vi "Clone Template Main.vi"() -> ()   [LabVIEW 2020, in "Template Tool.lvlib"]
uses:
  Template Tool.lvlib
  Queue Cluster.ctl
  Consumer State.ctl
  Consumer Data.ctl
  3a5bffab-33ac-43cc-aa37-910ccd41f3ad.vi
panel:
  in  "cancelling":string="\nCANCELLING\n\nThis may take a moment."
  out "Build Time (m:ss)":string
  in  "stop":bool
  out "message":string
  out "Progress":u8(slide) scale=0.0..100.0
  in  "start":bool
  in  "cancel":bool
  in  "Enter Destination Directory":path
  in  "Enter Custom Device Name":string="My New Comms"
  # "Instructions:\n1. Run this VI.\n2. Enter a Custom Device Name and Destination Directory.\n3. Press Start."
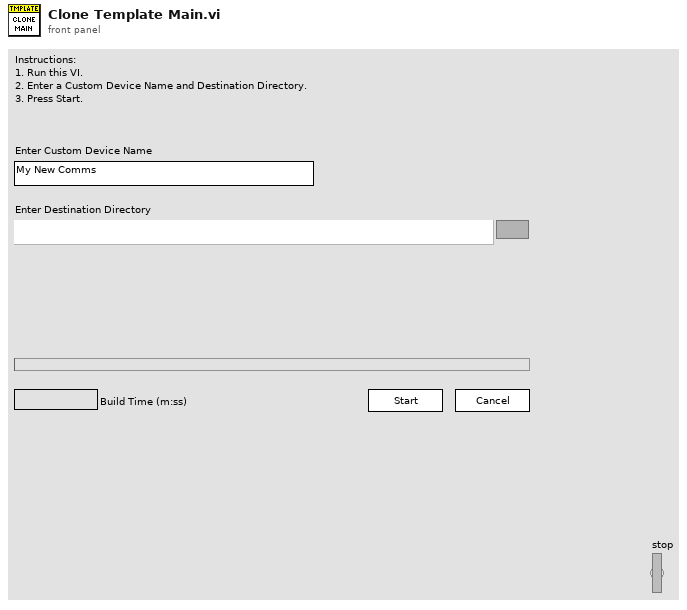
[diagram p1: front panel]
types:
  T1 = typedef "Template Tool.lvlib/Consumer Data.ctl" = cluster{"xml name":string, "CD name":string, "CD lvproj name":string, "CD support lvproj name":string, "custom device path":path, "progress":u8, "relative LVLIB folders":path[], "Public Docs CD path":path, "custom device lvproj path":path}
  T2 = typedef "Template Tool.lvlib/Queue Cluster.ctl" = cluster{"state":T3, "data":variant}
  T3 = typedef "Template Tool.lvlib/Consumer State.ctl" = enum16{"Init", "Cancel", "Copy Source", "Build Original Support PPLs", "Update Help Files", "Edit Page VIs Help CHM Constant", "Includes Folder AutoPopulate Off", "Replace VI & XML GUIDs", "Edit Paths in XML", "Edit CD Name in XML", "Edit VI Constants", "Edit Build Spec Destinations", "Delete Test Folders", "Create & Replace Support LVLIB Copies to Temp", "Create & Replace Support LVLIB Copies to Original", "Rename LVLIBS in Support LVPROJ File", "Update Support Build Specs and Build", "Replace Project PPLs", "Includes Folder AutoPopulate On", "Create & Replace LVLIB Copies to Temp", "Create & Replace LVLIB Copies to Original", "Rename LVLIBS in LVPROJ File", "Rename LLBs", "Update Build Specs and Build", "Finish"}
  T4 = cluster{"Enter Custom Device Name":string, "Enter Destination Directory":path}
  T5 = enum16{"Rename Original to Temp", "Rename Temp to Original"}
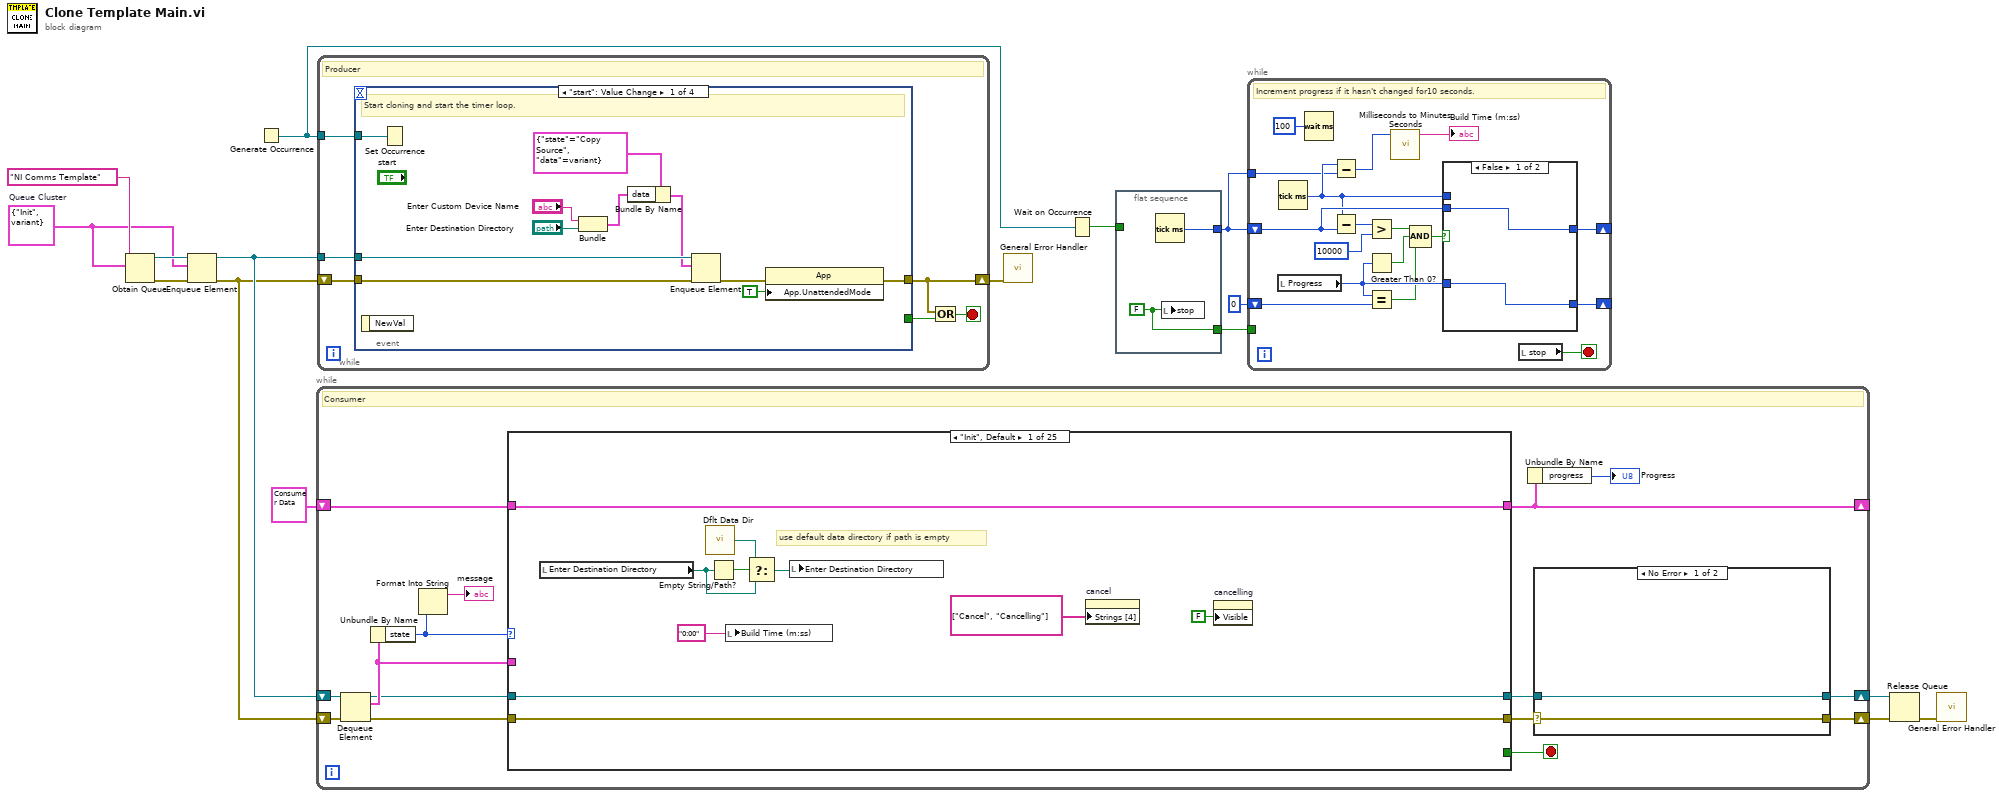
[diagram p0: block diagram]
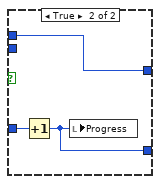
[diagram p2: hidden frame]
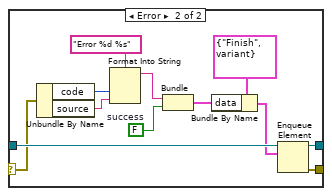
[diagram p3: hidden frame]
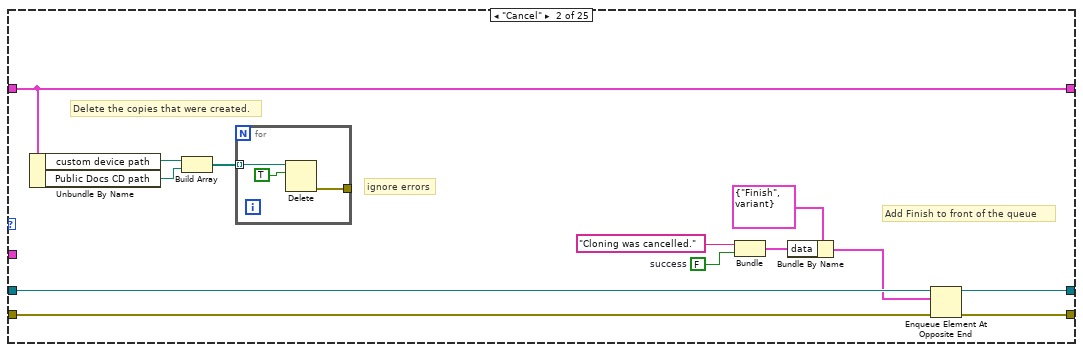
[diagram p4: hidden frame]
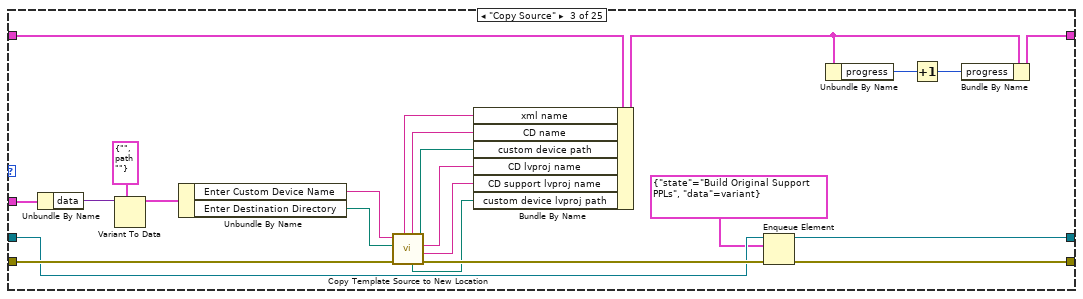
[diagram p5: hidden frame]
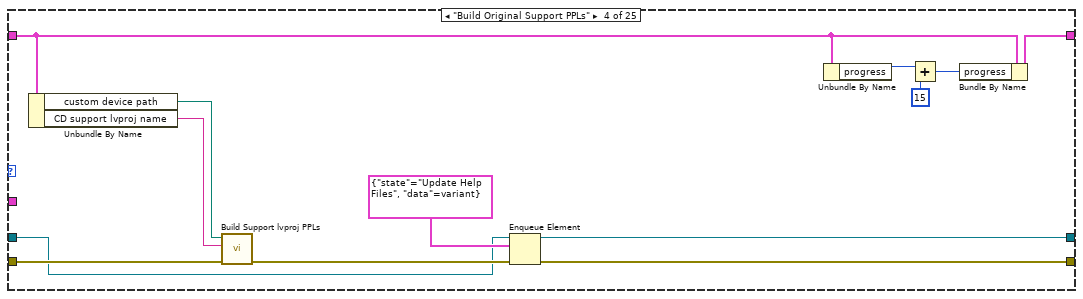
[diagram p6: hidden frame]
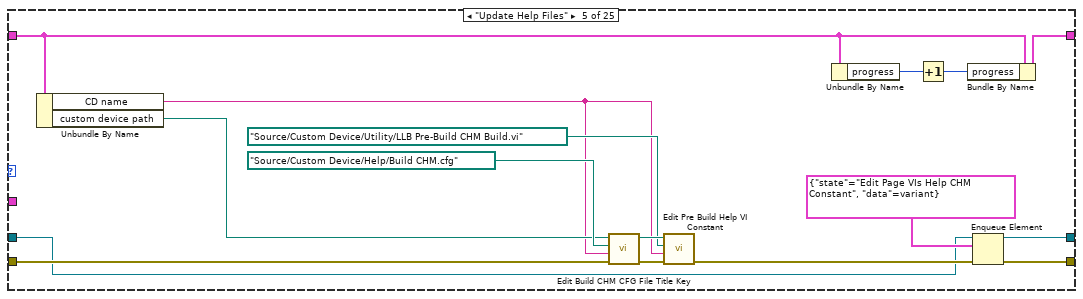
[diagram p7: hidden frame]
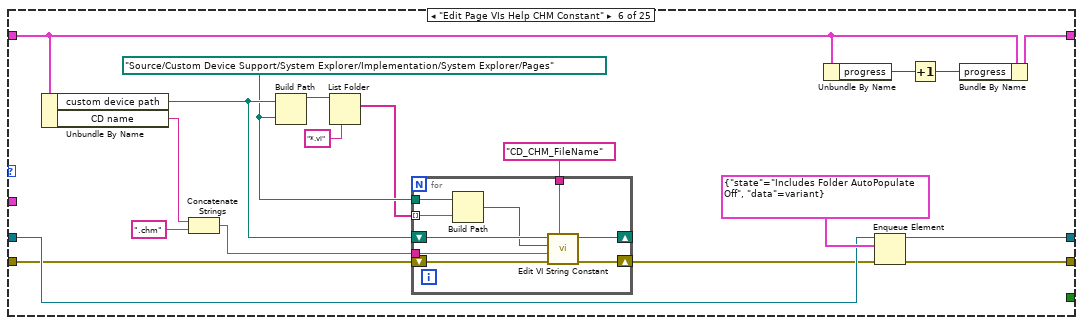
[diagram p8: hidden frame]
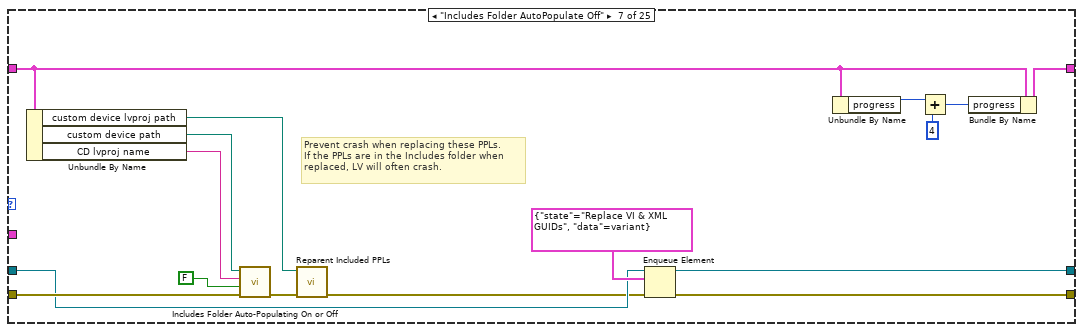
[diagram p9: hidden frame]
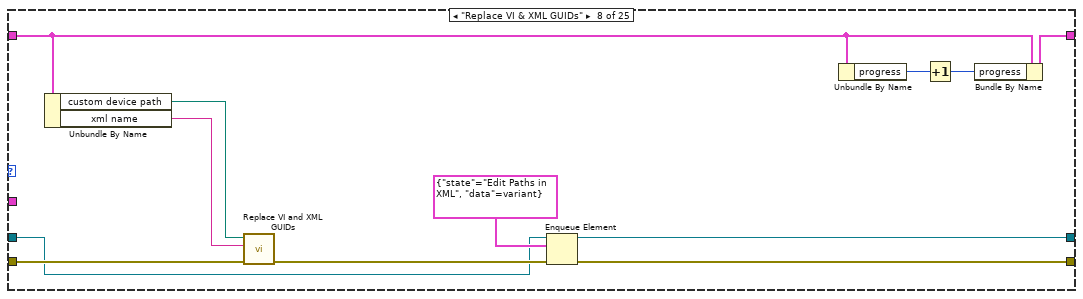
[diagram p10: hidden frame]
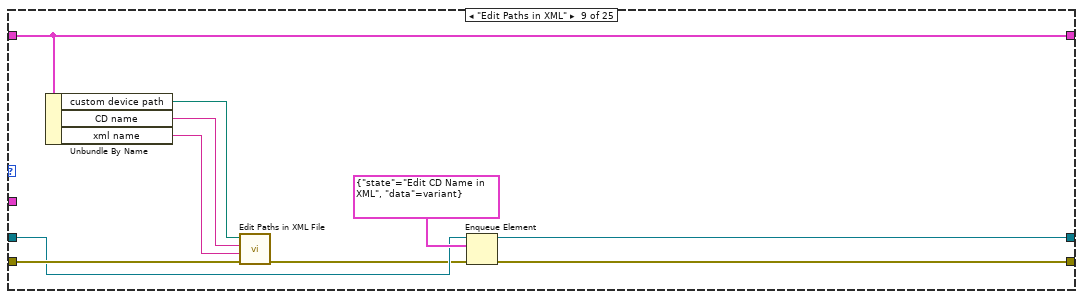
[diagram p11: hidden frame]
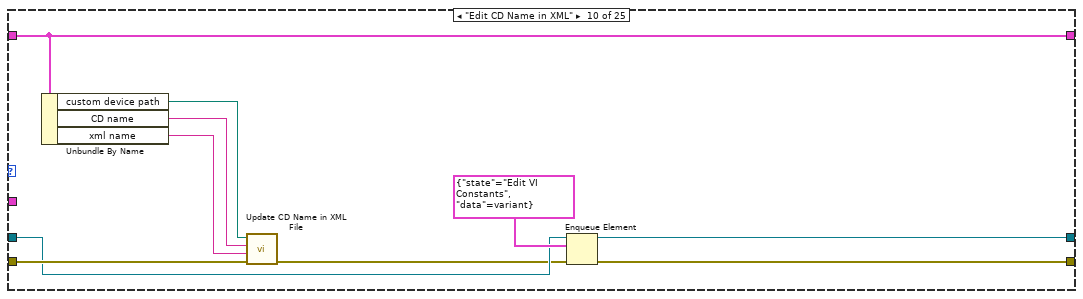
[diagram p12: hidden frame]
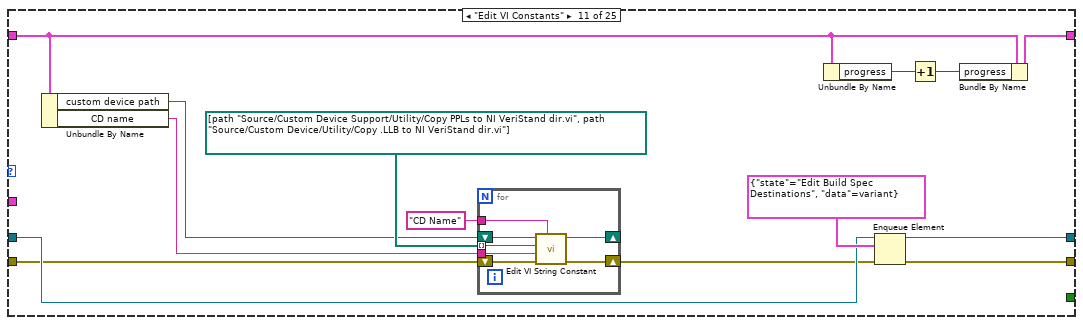
[diagram p13: hidden frame]
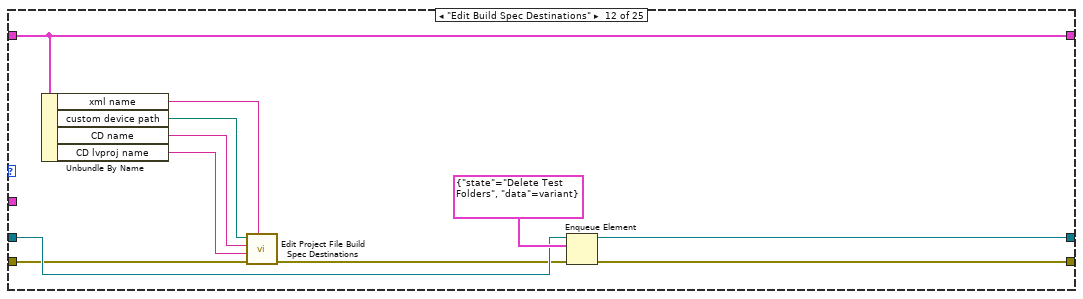
[diagram p14: hidden frame]
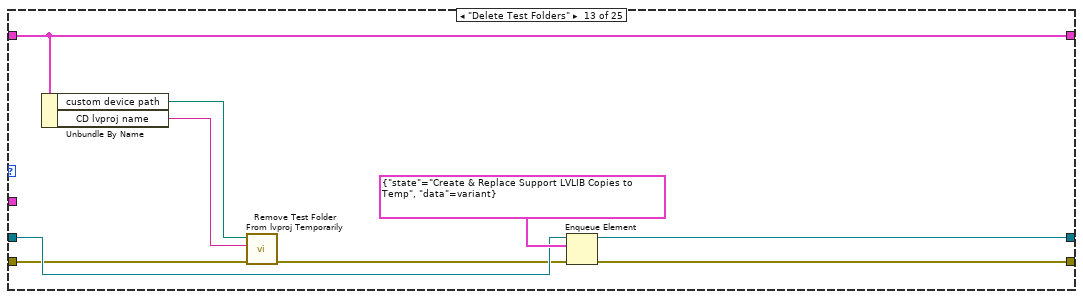
[diagram p15: hidden frame]
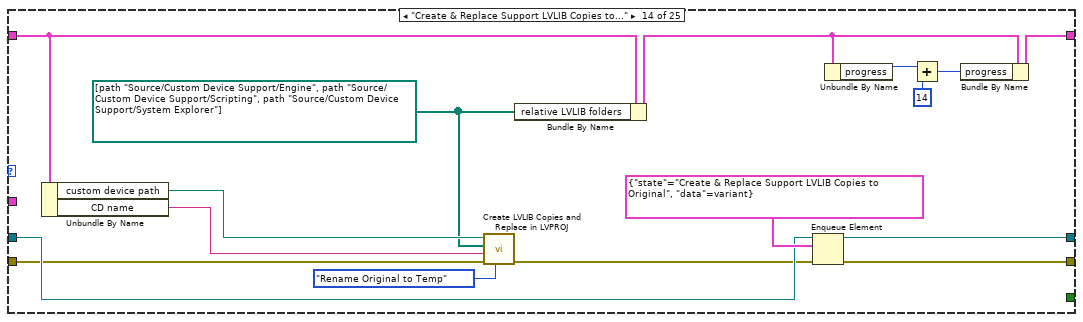
[diagram p16: hidden frame]
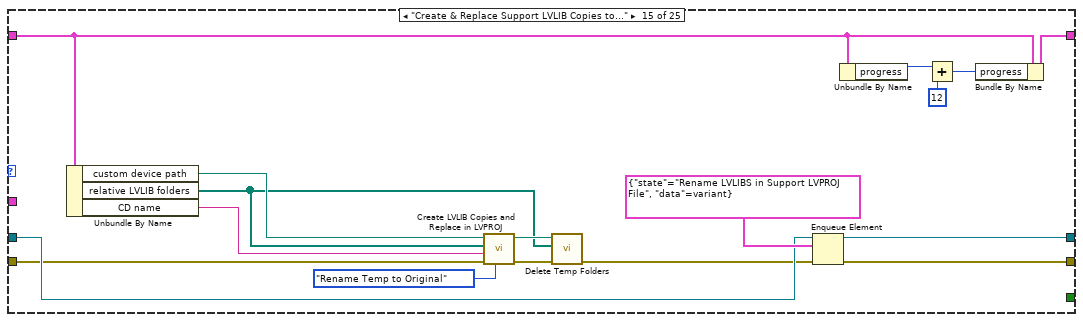
[diagram p17: hidden frame]
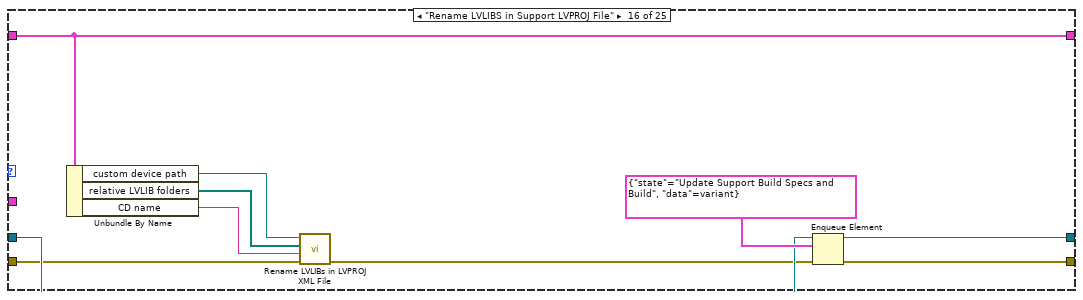
[diagram p18: hidden frame]
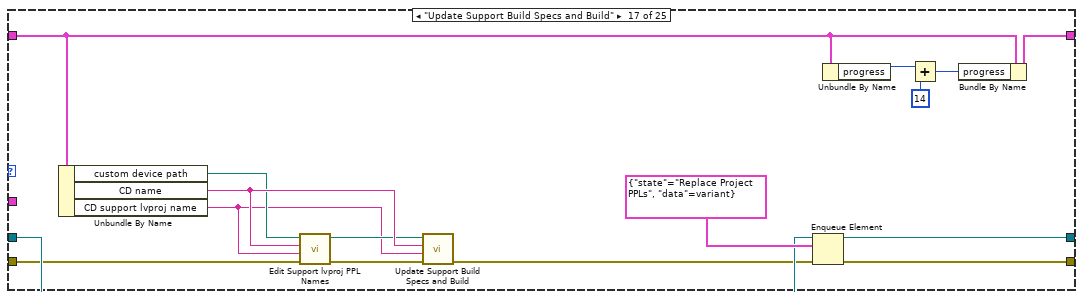
[diagram p19: hidden frame]
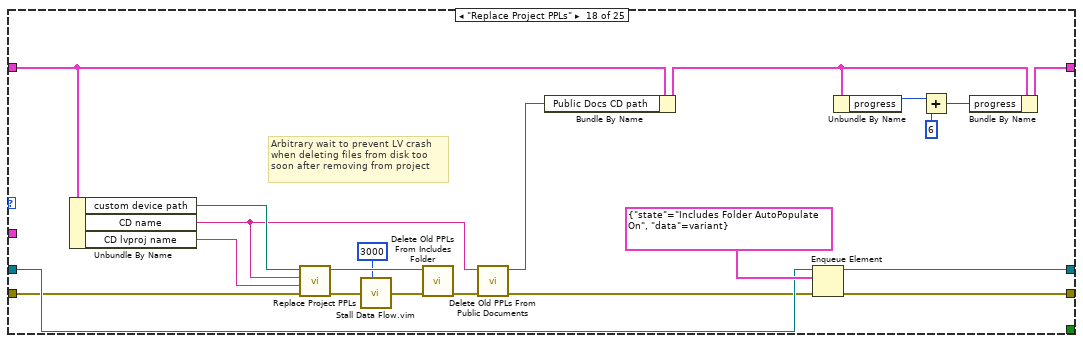
[diagram p20: hidden frame]
diagram:
  w12 = T2 {"state"=enum."Init", "data"=variant}  # Queue Cluster
  n1 = Obtain Queue(name (unnamed)="NI Comms Template", element data type=w12) -> (queue out=w15:refnum<queue>, error out=w14:errorcluster)  [unwired: 3 in, 1 out]
  n2 = Enqueue Element(queue=w15, element=w12, error in (no error)=w14) -> (queue out=w13:refnum<queue>, error out=w11:errorcluster)  [unwired: 1 in, 1 out]
  n3 = Generate Occurrence() -> (w2:refnum<k4>)
  n4 = while {
    shift-right: [w20] -> w9
    shift-left: w11 -> [w28]
    shift-right: [w23] -> _
    shift-left: T1 {"xml name"="", "CD name"="", "CD lvproj name"="", "CD support lvproj name"="", "custom device path"=path "", "progress"=0, "relative LVLIB folders"=[], "Public Docs CD path"=path "", "custom device lvproj path"=path ""} ("Consumer Data") -> [w29]
    shift-right: [w18] -> w8
    shift-left: w13 -> [w31]
    stop <- w17 stop-if-true
    # "Consumer"
    n5 = Dequeue Element(queue=w31, error in (no error)=w28) -> (queue out=w26:refnum<queue>, element=w30:T2, error out=w27:errorcluster)  [unwired: 1 in, 1 out]
    n6 = Unbundle By Name(w30) -> ("state"=w25:T3)
    n7 = Format Into String(w25) -> (resulting string=→"message":string)  [unwired: 3 in, 1 out]
    n8 = case shown="\"Init\", Default" w25 {
      tunnel: w30 -> [_ _ w94 _ _ _ _ _ _ _ _ _ _ _ _ _ _ _ _ _ _ _ _ _ w429]
      tunnel: [_ _ _ _ _ _ _ _ _ _ _ _ _ _ _ _ _ _ _ _ _ _ _ _ w420] -> w17
      tunnel: w27 -> [w50 w68 w93 w106 w119 w139 w167 w179 w188 w199 w209 w227 w236 w252 w270 w277 w295 w314 w334 w342 w368 w379 w389 w414 w418]
      tunnel: [w50 w67 w80 w103 w114 w137 w162 w174 w180 w190 w206 w221 w232 w246 w262 w279 w296 w317 w328 w348 w360 w381 w393 w415 w419] -> w21
      tunnel: w29 -> [w54 w58 w87 w98 w109 w134 w156 w169 w189 w198 w203 w231 w240 w256 w258 w280 w285 w308 w322 w354 w356 w373 w394 w410 w422]
      tunnel: [w54 w58 w73 w97 w108 w133 w155 w168 w189 w198 w202 w231 w240 w241 w257 w280 w284 w307 w321 w343 w355 w372 w394 w409 w422] -> w23
      tunnel: w26 -> [w55 w66 w79 w102 w112 w141 w161 w173 w183 w193 w212 w229 w238 w254 w272 w282 w298 w319 w327 w352 w370 w383 w396 w417 w427]
      tunnel: [w55 w65 w77 w101 w113 w140 w160 w172 w182 w192 w211 w228 w237 w253 w271 w281 w297 w318 w326 w351 w369 w382 w395 w416 w427] -> w19
      frame "Init", Default {
        # "use default data directory if path is empty"
        n9 = local read "Enter Destination Directory"() -> (w46:path)
        n10 = call <vilib>:"Dflt Data Dir.vi"() -> ("App:Default Data Directory"=w48:path)
        n11 = Empty String/Path?(string/path=w46) -> (empty?=w49:bool)
        n12 = local write "Build Time (m:ss)"("0:00" ("Build Time (m:s)")) -> ()
        n13 = Select(t=w48, s=w49, f=w46) -> (s? t:f=w47:path)
        n14 = local write "Enter Destination Directory"(w47) -> ()
        n15 = property on="cancel" class="Bool"("Strings [4]"=string[] ["Cancel", "Cancelling"]) -> ()  [unwired: 2 in, 2 out]
        n16 = property on="cancelling" class="Str"("Visible"=FALSE) -> ()  [unwired: 2 in, 2 out]
      }
      frame "Cancel" {
        w59 = FALSE  # success
        # "ignore errors"
        # "Add Finish to front of the queue"
        # "Delete the copies that were created."
        n17 = Unbundle By Name(w58) -> ("custom device path"=w64:path, "Public Docs CD path"=w56:path)
        n18 = Build Array(w64, w56) -> (w57:path[])
        n19 = for {
          tunnel: w57 -> [w71] mode=indexing
          tunnel: [w69] -> _
          n20 = Delete(path (use dialog)=w71, entire hierarchy (F)=TRUE) -> (error out=w69:errorcluster)  [unwired: 3 in, 2 out]
        }
        n21 = Bundle("dialog message"="Cloning was cancelled.", "success"=w59) -> (w60:cluster{"dialog message":string, "success":bool})  [unwired: 1 in]
        n22 = Bundle By Name(cluster=T2 {"state"=enum."Finish", "data"=variant} ("Queue Cluster"), "data"=w60) -> (w62:T2)
        n23 = Enqueue Element At Opposite End(queue=w66, element=w62, error in (no error)=w68) -> (queue out=w65:refnum<queue>, error out=w67:errorcluster)  [unwired: 1 in, 1 out]
      }
      frame "Copy Source" {
        n24 = Unbundle By Name(w94) -> ("data"=w92:variant)
        n25 = Variant To Data(type=T4 {"Enter Custom Device Name"="", "Enter Destination Directory"=path ""} ("output cluster"), Variant=w92) -> (data=w90:T4)  [unwired: 1 in, 1 out]
        n26 = Unbundle By Name(w90) -> ("Enter Custom Device Name"=w89:string, "Enter Destination Directory"=w88:path)
        n27 = call "Copy Template Source to New Location.vi"("error in"=w93, "destination directory (default data directory if empty)"=w88, "custom device name"=w89) -> ("error out"=w81:errorcluster, "CD support lvproj name"=w82:string, "CD lvproj name"=w83:string, "custom device path out"=w84:path, "custom device lvproj path"=w72:path, "CD name"=w85:string, "xml name"=w86:string)  [unwired: 2 in]
        n28 = Bundle By Name(cluster=w87, "xml name"=w86, "CD name"=w85, "custom device path"=w84, "CD lvproj name"=w83, "CD support lvproj name"=w82, "custom device lvproj path"=w72) -> (w74:T1)
        n29 = Enqueue Element(queue=w79, element=T2 {"state"=enum."Build Original Support PPLs", "data"=variant} ("Queue Cluster"), error in (no error)=w81) -> (queue out=w77:refnum<queue>, error out=w80:errorcluster)  [unwired: 1 in, 1 out]
        n30 = Unbundle By Name(w74) -> ("progress"=w76:u8)
        n31 = Increment(x=w76) -> (x+1=w75:u8)
        n32 = Bundle By Name(cluster=w74, "progress"=w75) -> (w73:T1)
      }
      frame "Build Original Support PPLs" {
        n33 = Unbundle By Name(w98) -> ("custom device path"=w107:path, "CD support lvproj name"=w100:string)
        n34 = call "Build Support lvproj PPLs.vi"("error in"=w106, "CD support lvproj name"=w100, "custom device path"=w107) -> ("error out"=w104:errorcluster)  [unwired: 7 in, 1 out]
        n35 = Enqueue Element(queue=w102, element=T2 {"state"=enum."Update Help Files", "data"=variant} ("Queue Cluster"), error in (no error)=w104) -> (queue out=w101:refnum<queue>, error out=w103:errorcluster)  [unwired: 1 in, 1 out]
        n36 = Unbundle By Name(w98) -> ("progress"=w96:u8)
        n37 = Add(x=w96, y=u8 15) -> (x+y=w99:u8)
        n38 = Bundle By Name(cluster=w98, "progress"=w99) -> (w97:T1)
      }
      frame "Update Help Files" {
        n39 = Unbundle By Name(w109) -> ("CD name"=w117:string, "custom device path"=w118:path)
        n40 = call "Edit Build CHM CFG File Title Key.vi"("error in"=w119, "CD name"=w117, "relative path of CFG file to edit"=path "Source/Custom Device/Help/Build CHM.cfg" ("relative path of VI to edit"), "custom device path"=w118) -> ("error out"=w121:errorcluster, "custom device path out"=w122:path)  [unwired: 6 in]
        n41 = call "Edit Pre Build Help VI Constant.vi"("error in"=w121, "CD name"=w117, "relative path of VI to edit"=path "Source/Custom Device/Utility/LLB Pre-Build CHM Build.vi", "custom device path"=w122) -> ("error out"=w115:errorcluster)  [unwired: 6 in, 1 out]
        n42 = Unbundle By Name(w109) -> ("progress"=w111:u8)
        n43 = Increment(x=w111) -> (x+1=w110:u8)
        n44 = Bundle By Name(cluster=w109, "progress"=w110) -> (w108:T1)
        n45 = Enqueue Element(queue=w112, element=T2 {"state"=enum."Edit Page VIs Help CHM Constant", "data"=variant} ("Queue Cluster"), error in (no error)=w115) -> (queue out=w113:refnum<queue>, error out=w114:errorcluster)  [unwired: 1 in, 1 out]
      }
      frame "Edit Page VIs Help CHM Constant" {
        w128 = path "Source/Custom Device Support/System Explorer/Implementation/System Explorer/Pages" ("name or relative path")
        n46 = Unbundle By Name(w134) -> ("custom device path"=w131:path, "CD name"=w124:string)
        n47 = Concatenate Strings(w124, ".chm" ("string")) -> (w125:string)
        n48 = Build Path(base path=w131, name or relative path=w128) -> (appended path=w130:path)
        n49 = List Folder(path=w130, pattern="*.vi") -> (filenames=w127:string[])  [unwired: 2 in, 3 out]
        n50 = for {
          shift-right: [w149] -> w138
          shift-left: w139 -> [w150]
          shift-right: [w148] -> _
          shift-left: w131 -> [w151]
          tunnel: w125 -> [w147]
          tunnel: "CD_CHM_FileName" ("CD name") -> [w146]
          tunnel: w128 -> [w145]
          tunnel: w127 -> [w144] mode=indexing
          n51 = Build Path(base path=w145, name or relative path=w144) -> (appended path=w143:path)
          n52 = call "Edit VI String Constant.vi"("string label"=w146, "error in"=w150, "new value"=w147, "relative path of VI to edit"=w143, "custom device path"=w151) -> ("error out"=w149:errorcluster, "custom device path out"=w148:path)  [unwired: 5 in]
        }
        n53 = Unbundle By Name(w134) -> ("progress"=w136:u8)
        n54 = Enqueue Element(queue=w141, element=T2 {"state"=enum."Includes Folder AutoPopulate Off", "data"=variant} ("Queue Cluster"), error in (no error)=w138) -> (queue out=w140:refnum<queue>, error out=w137:errorcluster)  [unwired: 1 in, 1 out]
        n55 = Increment(x=w136) -> (x+1=w135:u8)
        n56 = Bundle By Name(cluster=w134, "progress"=w135) -> (w133:T1)
      }
      frame "Includes Folder AutoPopulate Off" {
        # "Prevent crash when replacing these PPLs.\nIf the PPLs are in the Includes folder when\nreplaced, LV will often crash."
        n57 = Unbundle By Name(w156) -> ("custom device lvproj path"=w152:path, "custom device path"=w166:path, "CD lvproj name"=w165:string)
        n58 = call "Includes Folder Auto-Populating On or Off.vi"("error in"=w167, "auto-populate (ON)"=FALSE, "CD lvproj name"=w165, "custom device path"=w166) -> ("error out"=w154:errorcluster)  [unwired: 6 in, 1 out]
        n59 = call "Reparent Included PPLs.vi"("error in"=w154, "custom device project"=w152) -> ("error out"=w153:errorcluster)  [unwired: 9 in]
        n60 = Enqueue Element(queue=w161, element=T2 {"state"=enum."Replace VI & XML GUIDs", "data"=variant} ("Queue Cluster"), error in (no error)=w153) -> (queue out=w160:refnum<queue>, error out=w162:errorcluster)  [unwired: 1 in, 1 out]
        n61 = Unbundle By Name(w156) -> ("progress"=w158:u8)
        n62 = Add(x=w158, y=u8 4) -> (x+y=w159:u8)
        n63 = Bundle By Name(cluster=w156, "progress"=w159) -> (w155:T1)
      }
      frame "Replace VI & XML GUIDs" {
        n64 = Unbundle By Name(w169) -> ("custom device path"=w178:path, "xml name"=w177:string)
        n65 = call "Replace VI and XML GUIDs.vi"("error in"=w179, "xml name"=w177, "custom device path"=w178) -> ("error out"=w175:errorcluster)  [unwired: 7 in, 1 out]
        n66 = Enqueue Element(queue=w173, element=T2 {"state"=enum."Edit Paths in XML", "data"=variant} ("Queue Cluster"), error in (no error)=w175) -> (queue out=w172:refnum<queue>, error out=w174:errorcluster)  [unwired: 1 in, 1 out]
        n67 = Unbundle By Name(w169) -> ("progress"=w171:u8)
        n68 = Increment(x=w171) -> (x+1=w170:u8)
        n69 = Bundle By Name(cluster=w169, "progress"=w170) -> (w168:T1)
      }
      frame "Edit Paths in XML" {
        n70 = Unbundle By Name(w189) -> ("custom device path"=w187:path, "CD name"=w186:string, "xml name"=w185:string)
        n71 = call "Edit Paths in XML File.vi"("error in"=w188, "xml name"=w185, "CD name"=w186, "custom device path"=w187) -> ("error out"=w181:errorcluster)  [unwired: 5 in, 2 out]
        n72 = Enqueue Element(queue=w183, element=T2 {"state"=enum."Edit CD Name in XML", "data"=variant} ("Queue Cluster"), error in (no error)=w181) -> (queue out=w182:refnum<queue>, error out=w180:errorcluster)  [unwired: 1 in, 1 out]
      }
      frame "Edit CD Name in XML" {
        n73 = Unbundle By Name(w198) -> ("custom device path"=w197:path, "CD name"=w196:string, "xml name"=w195:string)
        n74 = call "Update CD Name in XML File.vi"("error in"=w199, "xml name"=w195, "CD name"=w196, "custom device path"=w197) -> ("error out"=w191:errorcluster)  [unwired: 6 in, 1 out]
        n75 = Enqueue Element(queue=w193, element=T2 {"state"=enum."Edit VI Constants", "data"=variant} ("Queue Cluster"), error in (no error)=w191) -> (queue out=w192:refnum<queue>, error out=w190:errorcluster)  [unwired: 1 in, 1 out]
      }
      frame "Edit VI Constants" {
        n76 = Unbundle By Name(w203) -> ("custom device path"=w208:path, "CD name"=w201:string)
        n77 = for {
          shift-right: [w218] -> w207
          shift-left: w209 -> [w219]
          tunnel: path[] [path "Source/Custom Device Support/Utility/Copy PPLs to NI VeriStand dir.vi", path "Source/Custom Device/Utility/Copy .LLB to NI VeriStand dir.vi"] -> [w217] mode=indexing
          shift-right: [w216] -> _
          shift-left: w208 -> [w220]
          tunnel: w201 -> [w215]
          tunnel: "CD Name" ("CD name") -> [w214]
          n78 = call "Edit VI String Constant.vi"("string label"=w214, "error in"=w219, "new value"=w215, "relative path of VI to edit"=w217, "custom device path"=w220) -> ("error out"=w218:errorcluster, "custom device path out"=w216:path)  [unwired: 5 in]
        }
        n79 = Unbundle By Name(w203) -> ("progress"=w205:u8)
        n80 = Enqueue Element(queue=w212, element=T2 {"state"=enum."Edit Build Spec Destinations", "data"=variant} ("Queue Cluster"), error in (no error)=w207) -> (queue out=w211:refnum<queue>, error out=w206:errorcluster)  [unwired: 1 in, 1 out]
        n81 = Increment(x=w205) -> (x+1=w204:u8)
        n82 = Bundle By Name(cluster=w203, "progress"=w204) -> (w202:T1)
      }
      frame "Edit Build Spec Destinations" {
        n83 = Unbundle By Name(w231) -> ("xml name"=w226:string, "custom device path"=w225:path, "CD name"=w224:string, "CD lvproj name"=w223:string)
        n84 = call "Edit Project File Build Spec Destinations.vi"("xml name"=w226, "error in"=w227, "CD lvproj name"=w223, "CD name"=w224, "custom device path"=w225) -> ("error out"=w222:errorcluster)  [unwired: 5 in, 1 out]
        n85 = Enqueue Element(queue=w229, element=T2 {"state"=enum."Delete Test Folders", "data"=variant} ("Queue Cluster"), error in (no error)=w222) -> (queue out=w228:refnum<queue>, error out=w221:errorcluster)  [unwired: 1 in, 1 out]
      }
      frame "Delete Test Folders" {
        n86 = Unbundle By Name(w240) -> ("custom device path"=w235:path, "CD lvproj name"=w234:string)
        n87 = call "Remove Test Folder From lvproj Temporarily.vi"("error in"=w236, "CD lvproj name"=w234, "custom device path"=w235) -> ("error out"=w233:errorcluster)  [unwired: 7 in, 1 out]
        n88 = Enqueue Element(queue=w238, element=T2 {"state"=enum."Create & Replace Support LVLIB Copies to Temp", "data"=variant} ("Queue Cluster"), error in (no error)=w233) -> (queue out=w237:refnum<queue>, error out=w232:errorcluster)  [unwired: 1 in, 1 out]
      }
      frame "Create & Replace Support LVLIB Copies to Temp" {
        w249 = path[] [path "Source/Custom Device Support/Engine", path "Source/Custom Device Support/Scripting", path "Source/Custom Device Support/System Explorer"] ("relative path of LVLIB folders")
        n89 = Unbundle By Name(w256) -> ("custom device path"=w251:path, "CD name"=w250:string)
        n90 = call "Create LVLIB Copies and Replace in LVPROJ.vi"("copy"=T5."Rename Original to Temp", "error in"=w252, "CD name"=w250, "relative path of LVLIB folders"=w249, "custom device path"=w251) -> ("error out"=w247:errorcluster)  [unwired: 5 in, 1 out]
        n91 = Bundle By Name(cluster=w256, "relative LVLIB folders"=w249) -> (w242:T1)
        n92 = Enqueue Element(queue=w254, element=T2 {"state"=enum."Create & Replace Support LVLIB Copies to Original", "data"=variant} ("Queue Cluster"), error in (no error)=w247) -> (queue out=w253:refnum<queue>, error out=w246:errorcluster)  [unwired: 1 in, 1 out]
        n93 = Unbundle By Name(w242) -> ("progress"=w244:u8)
        n94 = Add(x=w244, y=u8 14) -> (x+y=w245:u8)
        n95 = Bundle By Name(cluster=w242, "progress"=w245) -> (w241:T1)
      }
      frame "Create & Replace Support LVLIB Copies to Original" {
        n96 = Unbundle By Name(w258) -> ("custom device path"=w267:path, "relative LVLIB folders"=w264:path[], "CD name"=w269:string)
        n97 = call "Create LVLIB Copies and Replace in LVPROJ.vi"("copy"=T5."Rename Temp to Original", "error in"=w270, "CD name"=w269, "relative path of LVLIB folders"=w264, "custom device path"=w267) -> ("error out"=w266:errorcluster, "custom device path out"=w265:path)  [unwired: 5 in]
        n98 = call "Delete Temp Folders.vi"("error in"=w266, "relative path of LVLIB folders"=w264, "custom device path"=w265) -> ("error out"=w263:errorcluster)  [unwired: 7 in, 1 out]
        n99 = Enqueue Element(queue=w272, element=T2 {"state"=enum."Rename LVLIBS in Support LVPROJ File", "data"=variant} ("Queue Cluster"), error in (no error)=w263) -> (queue out=w271:refnum<queue>, error out=w262:errorcluster)  [unwired: 1 in, 1 out]
        n100 = Unbundle By Name(w258) -> ("progress"=w260:u8)
        n101 = Add(x=w260, y=u8 12) -> (x+y=w261:u8)
        n102 = Bundle By Name(cluster=w258, "progress"=w261) -> (w257:T1)
      }
      frame "Rename LVLIBS in Support LVPROJ File" {
        n103 = Unbundle By Name(w280) -> ("custom device path"=w276:path, "relative LVLIB folders"=w275:path[], "CD name"=w274:string)
        n104 = call "Rename LVLIBs in LVPROJ XML File.vi"("error in"=w277, "CD name"=w274, "relative path of LVLIB folders"=w275, "custom device path"=w276) -> ("error out"=w278:errorcluster)  [unwired: 6 in, 1 out]
        n105 = Enqueue Element(queue=w282, element=T2 {"state"=enum."Update Support Build Specs and Build", "data"=variant} ("Queue Cluster"), error in (no error)=w278) -> (queue out=w281:refnum<queue>, error out=w279:errorcluster)  [unwired: 1 in, 1 out]
      }
      frame "Update Support Build Specs and Build" {
        n106 = Unbundle By Name(w285) -> ("custom device path"=w291:path, "CD name"=w292:string, "CD support lvproj name"=w289:string)
        n107 = call "Edit Support lvproj PPL Names.vi"("error in"=w295, "CD support lvproj name"=w289, "CD name"=w292, "custom device path"=w291) -> ("error out"=w294:errorcluster, "custom device path out"=w290:path)  [unwired: 6 in]
        n108 = call "Update Support Build Specs and Build.vi"("error in"=w294, "CD support lvproj name"=w289, "CD name"=w292, "custom device path"=w290) -> ("error out"=w293:errorcluster)  [unwired: 6 in, 1 out]
        n109 = Enqueue Element(queue=w298, element=T2 {"state"=enum."Replace Project PPLs", "data"=variant} ("Queue Cluster"), error in (no error)=w293) -> (queue out=w297:refnum<queue>, error out=w296:errorcluster)  [unwired: 1 in, 1 out]
        n110 = Unbundle By Name(w285) -> ("progress"=w287:u8)
        n111 = Add(x=w287, y=u8 14) -> (x+y=w288:u8)
        n112 = Bundle By Name(cluster=w285, "progress"=w288) -> (w284:T1)
      }
      frame "Replace Project PPLs" {
        # "Arbitrary wait to prevent LV crash\nwhen deleting files from disk too\nsoon after removing from project"
        n113 = Unbundle By Name(w308) -> ("custom device path"=w313:path, "CD name"=w304:string, "CD lvproj name"=w312:string)
        n114 = call "Replace Project PPLs.vi"("error in"=w314, "CD lvproj name"=w312, "CD name"=w304, "custom device path"=w313) -> ("error out"=w316:errorcluster, "custom device path out"=w315:path)  [unwired: 6 in]
        n115 = call "Stall Data Flow.vim"("value in"=w316, "milliseconds to wait"=u32 3000) -> ("value out"=w301:errorcluster)  [unwired: 1 out]
        n116 = call "Delete Old PPLs From Includes Folder.vi"("error in"=w301, "custom device path"=w315) -> ("error out"=w306:errorcluster)  [unwired: 8 in, 1 out]
        n117 = call "Delete Old PPLs From Public Documents.vi"("error in"=w306, "CD name"=w304) -> ("error out"=w305:errorcluster, "Public Documents CD path"=w302:path)  [unwired: 8 in]
        n118 = Bundle By Name(cluster=w308, "Public Docs CD path"=w302) -> (w303:T1)
        n119 = Enqueue Element(queue=w319, element=T2 {"state"=enum."Includes Folder AutoPopulate On", "data"=variant} ("Queue Cluster"), error in (no error)=w305) -> (queue out=w318:refnum<queue>, error out=w317:errorcluster)  [unwired: 1 in, 1 out]
        n120 = Unbundle By Name(w303) -> ("progress"=w310:u8)
        n121 = Add(x=w310, y=u8 6) -> (x+y=w311:u8)
        n122 = Bundle By Name(cluster=w303, "progress"=w311) -> (w307:T1)
      }
      frame "Includes Folder AutoPopulate On" {
        n123 = Unbundle By Name(w322) -> ("custom device path"=w333:path, "CD lvproj name"=w332:string)
        n124 = call "Includes Folder Auto-Populating On or Off.vi"("error in"=w334, "auto-populate (ON)"=TRUE, "CD lvproj name"=w332, "custom device path"=w333) -> ("error out"=w329:errorcluster)  [unwired: 6 in, 1 out]
        n125 = Enqueue Element(queue=w327, element=T2 {"state"=enum."Create & Replace LVLIB Copies to Temp", "data"=variant} ("Queue Cluster"), error in (no error)=w329) -> (queue out=w326:refnum<queue>, error out=w328:errorcluster)  [unwired: 1 in, 1 out]
        n126 = Unbundle By Name(w322) -> ("progress"=w324:u8)
        n127 = Add(x=w324, y=u8 3) -> (x+y=w325:u8)
        n128 = Bundle By Name(cluster=w322, "progress"=w325) -> (w321:T1)
      }
      frame "Create & Replace LVLIB Copies to Temp" {
        w350 = path[] [path "Source/Custom Device/Shared", path "Source/Custom Device/System Explorer", path "Source/Custom Device/Engine"] ("relative path of LVLIB folders")
        n129 = Unbundle By Name(w354) -> ("custom device path"=w338:path, "CD name"=w336:string, "custom device lvproj path"=w337:path)
        n130 = call "Create Temporary Duplicate Project.vi"("error in"=w342, "project path"=w337) -> ("error out"=w341:errorcluster, "temp project path"=w339:path)  [unwired: 8 in]
        n131 = call "Create LVLIB Copies and Replace in LVPROJ.vi"("copy"=T5."Rename Original to Temp", "error in"=w341, "CD name"=w336, "relative path of LVLIB folders"=w350, "custom device path"=w338) -> ("error out"=w340:errorcluster)  [unwired: 5 in, 1 out]
        n132 = Bundle By Name(cluster=w354, "relative LVLIB folders"=w350) -> (w344:T1)
        n133 = call "Restore Build Specs After Replace.vi"("error in"=w340, "temporary project"=w339, "custom device project"=w337) -> ("error out"=w335:errorcluster)  [unwired: 8 in]
        n134 = Enqueue Element(queue=w352, element=T2 {"state"=enum."Create & Replace LVLIB Copies to Original", "data"=variant} ("Queue Cluster"), error in (no error)=w335) -> (queue out=w351:refnum<queue>, error out=w348:errorcluster)  [unwired: 1 in, 1 out]
        n135 = Unbundle By Name(w344) -> ("progress"=w346:u8)
        n136 = Add(x=w346, y=u8 9) -> (x+y=w347:u8)
        n137 = Bundle By Name(cluster=w344, "progress"=w347) -> (w343:T1)
      }
      frame "Create & Replace LVLIB Copies to Original" {
        n138 = Unbundle By Name(w356) -> ("custom device path"=w365:path, "relative LVLIB folders"=w362:path[], "CD name"=w367:string)
        n139 = call "Create LVLIB Copies and Replace in LVPROJ.vi"("copy"=T5."Rename Temp to Original", "error in"=w368, "CD name"=w367, "relative path of LVLIB folders"=w362, "custom device path"=w365) -> ("error out"=w364:errorcluster, "custom device path out"=w363:path)  [unwired: 5 in]
        n140 = call "Delete Temp Folders.vi"("error in"=w364, "relative path of LVLIB folders"=w362, "custom device path"=w363) -> ("error out"=w361:errorcluster)  [unwired: 7 in, 1 out]
        n141 = Enqueue Element(queue=w370, element=T2 {"state"=enum."Rename LVLIBS in LVPROJ File", "data"=variant} ("Queue Cluster"), error in (no error)=w361) -> (queue out=w369:refnum<queue>, error out=w360:errorcluster)  [unwired: 1 in, 1 out]
        n142 = Unbundle By Name(w356) -> ("progress"=w358:u8)
        n143 = Add(x=w358, y=u8 9) -> (x+y=w359:u8)
        n144 = Bundle By Name(cluster=w356, "progress"=w359) -> (w355:T1)
      }
      frame "Rename LVLIBS in LVPROJ File" {
        n145 = Unbundle By Name(w373) -> ("custom device path"=w378:path, "relative LVLIB folders"=w377:path[], "CD name"=w376:string)
        n146 = call "Rename LVLIBs in LVPROJ XML File.vi"("error in"=w379, "CD name"=w376, "relative path of LVLIB folders"=w377, "custom device path"=w378) -> ("error out"=w380:errorcluster)  [unwired: 6 in, 1 out]
        n147 = Enqueue Element(queue=w383, element=T2 {"state"=enum."Rename LLBs", "data"=variant} ("Queue Cluster"), error in (no error)=w380) -> (queue out=w382:refnum<queue>, error out=w381:errorcluster)  [unwired: 1 in, 1 out]
        n148 = Unbundle By Name(w373) -> ("progress"=w375:u8)
        n149 = Increment(x=w375) -> (x+1=w374:u8)
        n150 = Bundle By Name(cluster=w373, "progress"=w374) -> (w372:T1)
      }
      frame "Rename LLBs" {
        n151 = Unbundle By Name(w394) -> ("custom device path"=w388:path, "CD name"=w387:string, "xml name"=w385:string, "CD lvproj name"=w386:string)
        n152 = call "Rename Configuration LLB in LVPROJ.vi"("error in"=w389, "CD lvproj name"=w386, "CD name"=w387, "custom device path"=w388) -> ("error out"=w392:errorcluster, "custom device path out"=w390:path)  [unwired: 6 in]
        n153 = call "Rename LLBs in XML File.vi"("error in"=w392, "xml name"=w385, "CD name"=w387, "custom device path"=w390) -> ("error out"=w391:errorcluster)  [unwired: 6 in, 1 out]
        n154 = Enqueue Element(queue=w396, element=T2 {"state"=enum."Update Build Specs and Build", "data"=variant} ("Queue Cluster"), error in (no error)=w391) -> (queue out=w395:refnum<queue>, error out=w393:errorcluster)  [unwired: 1 in, 1 out]
      }
      frame "Update Build Specs and Build" {
        w401 = TRUE  # success
        n155 = Unbundle By Name(w410) -> ("custom device path"=w406:path, "custom device lvproj path"=w398:path, "CD name"=w399:string)
        n156 = call "Update Build Specs and Build.vi"("error in"=w414, "CD name"=w399, "custom device lvproj path"=w398) -> ("error out"=w400:errorcluster)  [unwired: 7 in, 1 out]
        n157 = Format Into String(format string=" %s", initial string="Cloning was successful and located at:" ("dialog message"), w406) -> (resulting string=w403:string)  [unwired: 1 in, 1 out]
        n158 = Bundle(w403, "success"=w401) -> (w402:cluster{string, "success":bool})  [unwired: 1 in]
        n159 = Bundle By Name(cluster=T2 {"state"=enum."Finish", "data"=variant} ("Queue Cluster"), "data"=w402) -> (w407:T2)
        n160 = Enqueue Element(queue=w417, element=w407, error in (no error)=w400) -> (queue out=w416:refnum<queue>, error out=w415:errorcluster)  [unwired: 1 in, 1 out]
        n161 = Unbundle By Name(w410) -> ("progress"=w412:u8)
        n162 = Add(x=w412, y=u8 9) -> (x+y=w413:u8)
        n163 = Bundle By Name(cluster=w410, "progress"=w413) -> (w409:T1)
      }
      frame "Finish" {
        w420 = TRUE
        n164 = flat-sequence {
          tunnel: [cluster{"dialog message":string, "success":bool} {"dialog message"="", "success"=FALSE} ("output cluster")] -> w426
          frame #0 {
            w430 = FALSE ("Application:Unattended Mode")
            # "Run this code prior to the dialog and ignore errors."
            n165 = property class="App"("App.UnattendedMode"=w430) -> ()  [unwired: 2 in, 2 out]
            n166 = property on="cancelling" class="Str"("Visible"=w430) -> ()  [unwired: 2 in, 2 out]
            n167 = call <vilib>:"Unset Busy.vi"() -> ()  [unwired: 11 in, 1 out]
          }
        }
        n168 = Unbundle By Name(w429) -> ("data"=w428:variant)
        n169 = Variant To Data(error in=w418, type=w426, Variant=w428) -> (data=w425:cluster{"dialog message":string, "success":bool}, error out=w419:errorcluster)
        n170 = Unbundle By Name(w422) -> ("custom device path"=w421:path)
        n171 = Unbundle By Name(w425) -> ("dialog message"=w423:string, "success"=w424:bool)
        n172 = case shown="True" w424 {
          tunnel: w423 -> [w432 w435]
          tunnel: w421 -> [_ w436]
          frame False {
            n173 = One Button Dialog(message=w432) -> ()  [unwired: 1 in, 1 out]
          }
          frame True {
            n174 = Two Button Dialog(message=w435, 1:"Done" ("F button name (\"Cancel\")"), 2:"Explore" ("F button name (\"Cancel\")")) -> (T button?=w437:bool)
            n175 = case shown="True" w437 {
              tunnel: w436 -> [_ w441]
              frame False {
              }
              frame True {
                n176 = call <vilib>:"System Exec.vi"("run minimized? (F)"=TRUE, "wait until completion? (T)"=FALSE, "working directory"=w441, "command line"="cmd /c start .") -> ()  [unwired: 4 in, 4 out]
              }
            }
          }
        }
        n177 = property on="stop" class="Bool (strict)"("Val(Sgnl)"=w420) -> ()  [unwired: 2 in, 2 out]
      }
    }
    n178 = Unbundle By Name(w23) -> ("progress"=→"Progress":u8)
    n179 = case shown="No Error" w21 {
      selector: w21 -> [w33 w41]
      tunnel: [w33 w43] -> w20
      tunnel: w19 -> [w32 w45]
      tunnel: [w32 w44] -> w18
      frame No Error {
      }
      frame Error {
        w34 = FALSE  # success
        n180 = Unbundle By Name(w41) -> ("code"=w40:i32, "source"=w39:string)
        n181 = Format Into String(format string="Error %d %s" ("dialog message"), w40, w39) -> (resulting string=w37:string)  [unwired: 2 in, 1 out]
        n182 = Bundle(w37, "success"=w34) -> (w35:cluster{string, "success":bool})  [unwired: 1 in]
        n183 = Bundle By Name(cluster=T2 {"state"=enum."Finish", "data"=variant} ("Queue Cluster"), "data"=w35) -> (w36:T2)
        n184 = Enqueue Element(queue=w45, element=w36) -> (queue out=w44:refnum<queue>, error out=w43:errorcluster)  [unwired: 2 in, 1 out]
      }
    }
  }
  n185 = while {
    shift-right: [w443] -> w7
    shift-left: w11 -> [w446]
    tunnel: w13 -> [w447]
    tunnel: w2 -> [w442]
    stop <- w444 stop-if-true
    # "Producer"
    n186 = event shown="[0] \"start\": Value Change" {
      selector: _ -> [_ _ _ _]
      dyn-events: _ -> [_ _ _ _]
      timeout: _ -> [_ _ _ _]
      tunnel: w447 -> [w458 w467 _ _]
      tunnel: w446 -> [w457 w466 w468 w471]
      tunnel: [w450 w463 w468 w471] -> w443
      tunnel: [_ "cancel" _ "stop"] -> w445
      tunnel: w442 -> [w448 w462 _ _]
      event "start": Value Change {
        # "Start cloning and start the timer loop."
        n187 = event-data() -> ()  [unwired: 1 in, 1 out]
        n188 = Set Occurrence(w448) -> ()
        n189 = Bundle("Enter Custom Device Name"="Enter Custom Device Name", "Enter Destination Directory"="Enter Destination Directory") -> (w453:T4)  [unwired: 1 in]
        n190 = Bundle By Name(cluster=T2 {"state"=enum."Copy Source", "data"=variant} ("Queue Cluster"), "data"=w453) -> (w454:T2)
        n191 = Enqueue Element(queue=w458, element=w454, error in (no error)=w457) -> (error out=w451:errorcluster)  [unwired: 1 in, 2 out]
        n192 = property class="App"(error in=w451, "App.UnattendedMode"=TRUE ("Application:Unattended Mode")) -> (error out=w450:errorcluster)  [unwired: 1 in, 1 out]
      }
      event "cancel": Value Change {
        # "This is released in the Finish case."
        # "Calls Cancel case to delete copies that were created."
        n193 = event-data() -> ("NewVal"=w459:bool)  [unwired: 1 in]
        n194 = Set Occurrence(w462) -> ()
        n195 = Enqueue Element At Opposite End(queue=w467, element=T2 {"state"=enum."Cancel", "data"=variant} ("Queue Cluster"), error in (no error)=w466) -> (error out=w461:errorcluster)  [unwired: 1 in, 2 out]
        n196 = property on="cancelling" class="Str"(error in=w461, "Visible"=w459) -> (error out=w460:errorcluster)  [unwired: 1 in, 1 out]
        n197 = call <vilib>:"Set Busy.vi"("error in (no error)"=w460) -> ("error out"=w463:errorcluster)  [unwired: 9 in, 1 out]
      }
      event Panel Close? {
        n198 = event-data() -> ()  [unwired: 1 in, 2 out]
        n199 = event-data("Discard?"=TRUE) -> ()  [unwired: 1 in, 1 out]
      }
      event "stop": Value Change {
        # "This gets called via a Val(Sgnl) call in the Consumer Finish case."
        n200 = event-data() -> ()  [unwired: 1 in, 1 out]
      }
    }
    n201 = Or(x=w443, y=w445) -> (x .or. y?=w444:bool)
  }
  n202 = call <vilib>:"General Error Handler.vi"("error in (no error)"=w7) -> ()  [unwired: 10 in, 5 out]
  n203 = Wait on Occurrence(2:w2) -> (0:w1:bool)  [unwired: 2 in]
  n204 = flat-sequence {
    tunnel: [w473] -> w6
    tunnel: [w472] -> w4
    tunnel: w1 -> [_]
    frame #0 {
      w473 = FALSE ("progress loop")
      n205 = Tick Count (ms)() -> (millisecond timer value=w472:u32)
      n206 = local write "stop"(w473) -> ()
    }
  }
  n207 = while {
    shift-right: [w485] -> _
    shift-left: w4 -> [w484]
    tunnel: w6 -> [_]
    shift-right: [w480] -> _
    shift-left: u8 0 ("Progress") -> [w483]
    tunnel: w4 -> [w476]
    stop <- w479 stop-if-true
    # "Increment progress if it hasn't changed for10 seconds."
    n208 = local read "Progress"() -> (w482:u8)
    n209 = Tick Count (ms)() -> (millisecond timer value=w477:u32)
    n210 = Wait (ms)(milliseconds to wait=u32 100) -> ()  [unwired: 1 out]
    n211 = Subtract(x=w477, y=w476) -> (x-y=w475:u32)
    n212 = Subtract(x=w477, y=w484) -> (x-y=w478:u32)
    n213 = Greater?(x=w478, y=u32 10000) -> (0:w488:bool)
    n214 = Greater Than 0?(x=w482) -> (x > 0?=w487:bool)
    n215 = Equal?(x=w482, y=w483) -> (x = y?=w481:bool)
    n216 = call "Milliseconds to Minutes Seconds.vi"("milliseconds"=w475) -> ("minutes:seconds"=→"Build Time (m:ss)":string)  [unwired: 10 in]
    n217 = Compound Arithmetic op=AND(w488, w487, w481) -> (w486:bool)
    n218 = case shown="False" w486 {
      tunnel: w482 -> [w491 w495]
      tunnel: [w492 w494] -> w485
      tunnel: w477 -> [_ w494]
      tunnel: w484 -> [w492 _]
      tunnel: [w491 w493] -> w480
      frame False {
      }
      frame True {
        n219 = Increment(x=w495) -> (x+1=w493:u8)
        n220 = local write "Progress"(w493) -> ()
      }
    }
    n221 = local read "stop"() -> (w479:bool)
  }
  n222 = Release Queue(queue=w8, error in (no error)=w9) -> (error out=w3:errorcluster)  [unwired: 1 in, 2 out]
  n223 = call <vilib>:"General Error Handler.vi"("error in (no error)"=w3) -> ()  [unwired: 10 in, 5 out]
